vi "Initialize Sequence Execution Tree.vi"(11 "UI Data in":refnum<class "Settings UI.lvclass">) -> (2 "Items to Add":T1(array[cluster]), 3 "UI Data out":refnum<class "Settings UI.lvclass">)   [LabVIEW 2020, in "Output Sequencer.lvlib" / "Settings UI.lvclass"]
uses:
  Settings UI.lvclass
  Types/Tree Index Enum.ctl
  Settings UI.lvclass/Settings UI.ctl
  Globals/Global Tree Data.vi
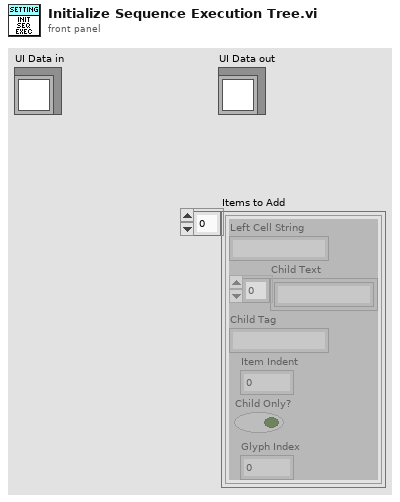
[diagram p1: front panel]
types:
  T1 = cluster{"Left Cell String":string, "Child Text":string[], "Child Tag":string, "Item Indent":i32, "Child Only?":bool, "Glyph Index":i32}[]
  T2 = typedef "Output Sequencer.lvlib/Settings UI.lvclass/Tree Index Enum.ctl" = enum16{"General Settings", "Num Steps", "Num Analog", "Num Digital", "Show Confirmation", "Interp Priority", "Adv Timing", "Enable Conditions", "Seq Execution", "Reset Test Start", "Only When Test", "Delay After Test", "Start condition", "Re-triggering", "Stop condition", "Stop After Cycles", "Stop Values", "Default Values", "Default Analog", "Default Digital", "Steps", "Step #", "Description", "Precondition", "Duration", "Mode", "Delay Between Vals", "Analog Values", "Digital Values", "Postcondition", "On True", "On False"}
  T3 = typedef "Output Sequencer.lvlib/Settings UI.lvclass/Tree Item Settings.ctl" = cluster{"Tree Label":string, "Indent Level":i32, "Data Type":T4, "Numeric Range":cluster{"Min":dbl, "Max":dbl, "Inc":dbl}, "Allowed Values":string[], "Default Value":string, "Description":string}
  T4 = typedef "Output Sequencer.lvlib/Settings UI.lvclass/Data Type.ctl" = i16
  T5 = cluster{"Left Cell String":string, "Child Text":string[], "Child Tag":string, "Item Indent":i32, "Child Only?":bool, "Glyph Index":i32}
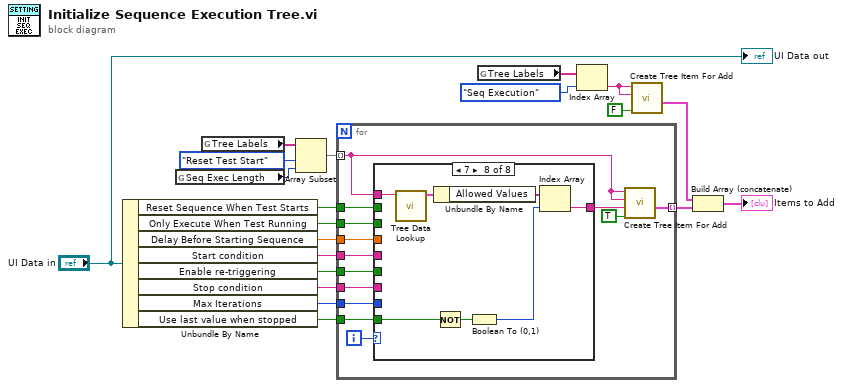
[diagram p0: block diagram]
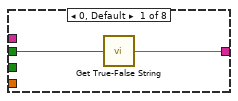
[diagram p2: hidden frame]
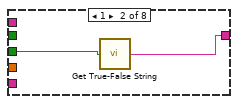
[diagram p3: hidden frame]
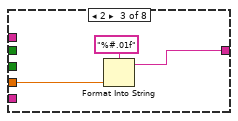
[diagram p4: hidden frame]
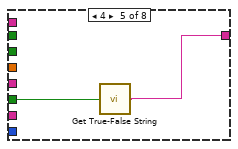
[diagram p6: hidden frame]
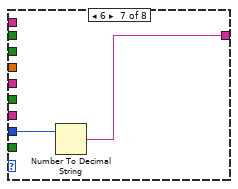
[diagram p8: hidden frame]
diagram:
  n1 = Unbundle By Name("UI Data in") -> ("Reset Sequence When Test Starts"=w10:bool, "Only Execute When Test Running"=w9:bool, "Delay Before Starting Sequence"=w18:dbl, "Start condition"=w5:string, "Enable re-triggering"=w4:bool, "Stop condition"=w3:string, "Max Iterations"=w6:u32, "Use last value when stopped"=w11:bool)
  n2 = global read "Global Tree Data.vi" "Seq Exec Length"() -> (w15:i32)
  n3 = global read "Global Tree Data.vi" "Tree Labels"() -> (w17:string[])
  n4 = Array Subset(array=w17, index=Tree_Index_Enum."Reset Test Start" ("Tree Index Enum"), length=w15) -> (w16:string[])
  n5 = for {
    tunnel: w16 -> [w24] mode=indexing
    tunnel: w18 -> [w33]
    tunnel: w9 -> [w32]
    tunnel: w10 -> [w31]
    tunnel: [w29] -> w2 mode=indexing
    tunnel: w6 -> [w26]
    tunnel: w11 -> [w25]
    tunnel: w5 -> [w23]
    tunnel: w4 -> [w22]
    tunnel: w3 -> [w21]
    i -> [w30]
    n6 = case shown="7" w30 {
      tunnel: w33 -> [_ _ w39 _ _ _ _ _]
      tunnel: w32 -> [_ w37 _ _ _ _ _ _]
      tunnel: w31 -> [w35 _ _ _ _ _ _ _]
      tunnel: [w34 w36 w38 w41 w42 w44 w46 w47] -> w28
      tunnel: w26 -> [_ _ _ _ _ _ w45 _]
      tunnel: w25 -> [_ _ _ _ _ _ _ w51]
      tunnel: w24 -> [_ _ _ _ _ _ _ w53]
      tunnel: w23 -> [_ _ _ w41 _ _ _ _]
      tunnel: w22 -> [_ _ _ _ w43 _ _ _]
      tunnel: w21 -> [_ _ _ _ _ w44 _ _]
      frame 0, Default {
        n7 = call "Get True-False String.vi"("Input"=w35) -> ("True/False String"=w34:string)
      }
      frame 1 {
        n8 = call "Get True-False String.vi"("Input"=w37) -> ("True/False String"=w36:string)
      }
      frame 2 {
        n9 = Format Into String(format string="%#.01f", w39) -> (resulting string=w38:string)  [unwired: 2 in, 1 out]
      }
      frame 3 {
      }
      frame 4 {
        n10 = call "Get True-False String.vi"("Input"=w43) -> ("True/False String"=w42:string)
      }
      frame 5 {
      }
      frame 6 {
        n11 = Number To Decimal String(number=w45) -> (decimal integer string=w46:string)  [unwired: 1 in]
      }
      frame 7 {
        n12 = call "Tree Data Lookup.vi"("Tag in"=w53) -> ("Tree Data"=w52:T3)  [unwired: 5 in, 5 out]
        n13 = Unbundle By Name(w52) -> ("Allowed Values"=w49:string[])
        n14 = Not(x=w51) -> (.not. x?=w50:bool)
        n15 = Boolean To (0,1)(Boolean=w50) -> (0, 1=w48:i16)
        n16 = Index Array(array=w49, index=w48) -> (element=w47:string)
      }
    }
    n17 = call "Create Tree Item For Add.vi"("Child Only? (true)"=TRUE ("Child Only? (False)"), "Child Text"=w28, "Left Cell String"=w24, "Child Tag in"=w24) -> ("Item"=w29:T5)  [unwired: 6 in, 1 out]
  }
  n18 = global read "Global Tree Data.vi" "Tree Labels"() -> (w14:string[])
  n19 = Index Array(array=w14, index=Tree_Index_Enum."Seq Execution" ("Tree Index Enum")) -> (element=w13:string)
  n20 = call "Create Tree Item For Add.vi"("Child Only? (true)"=FALSE, "Left Cell String"=w13, "Child Tag in"=w13) -> ("Item"=w1:T5)  [unwired: 7 in, 1 out]
  n21 = Build Array (concatenate)(w1, w2) -> (→"Items to Add":T1)
  "UI Data out" <- "UI Data in"
